vi "BioFeedback3(AudioInput+CircularBuffer).vi"() -> ()   [LabVIEW 2016]
uses:
  <vilib>/Analysis/5stat.llb/RMS (DBL).vi
  <vilib>/Analysis/baseanly.llb/Mean (DBL).vi
  <vilib>/Analysis/NI_AALBase.lvlib
  <vilib>/Analysis/NI_AALPro.lvlib
panel:
  out "Thermometer":dbl(slide) scale=0.0..0.07
  out "Circular Buffer Waveform\nData":waveform(dbl)(graph)
  out "Circular Buffer Waveform":waveform(dbl)[](graph)
  in  "bufferSize":dbl
  in  "Sample Duration":dbl
  out "filetered rms":waveform(dbl)(graph)
  out "filetered RMS Value 2":dbl
  out "RMS":waveform(dbl)(graph)
  out "RMS Value":dbl
  out "filtered":waveform(dbl)(graph)
  out "filtered + positivepeaks":waveform(dbl)(graph)
  out "Peaks Waveform (OLD)":waveform(dbl)(graph)
  out "Raw Audio\nWaveform":waveform(dbl)(graph)
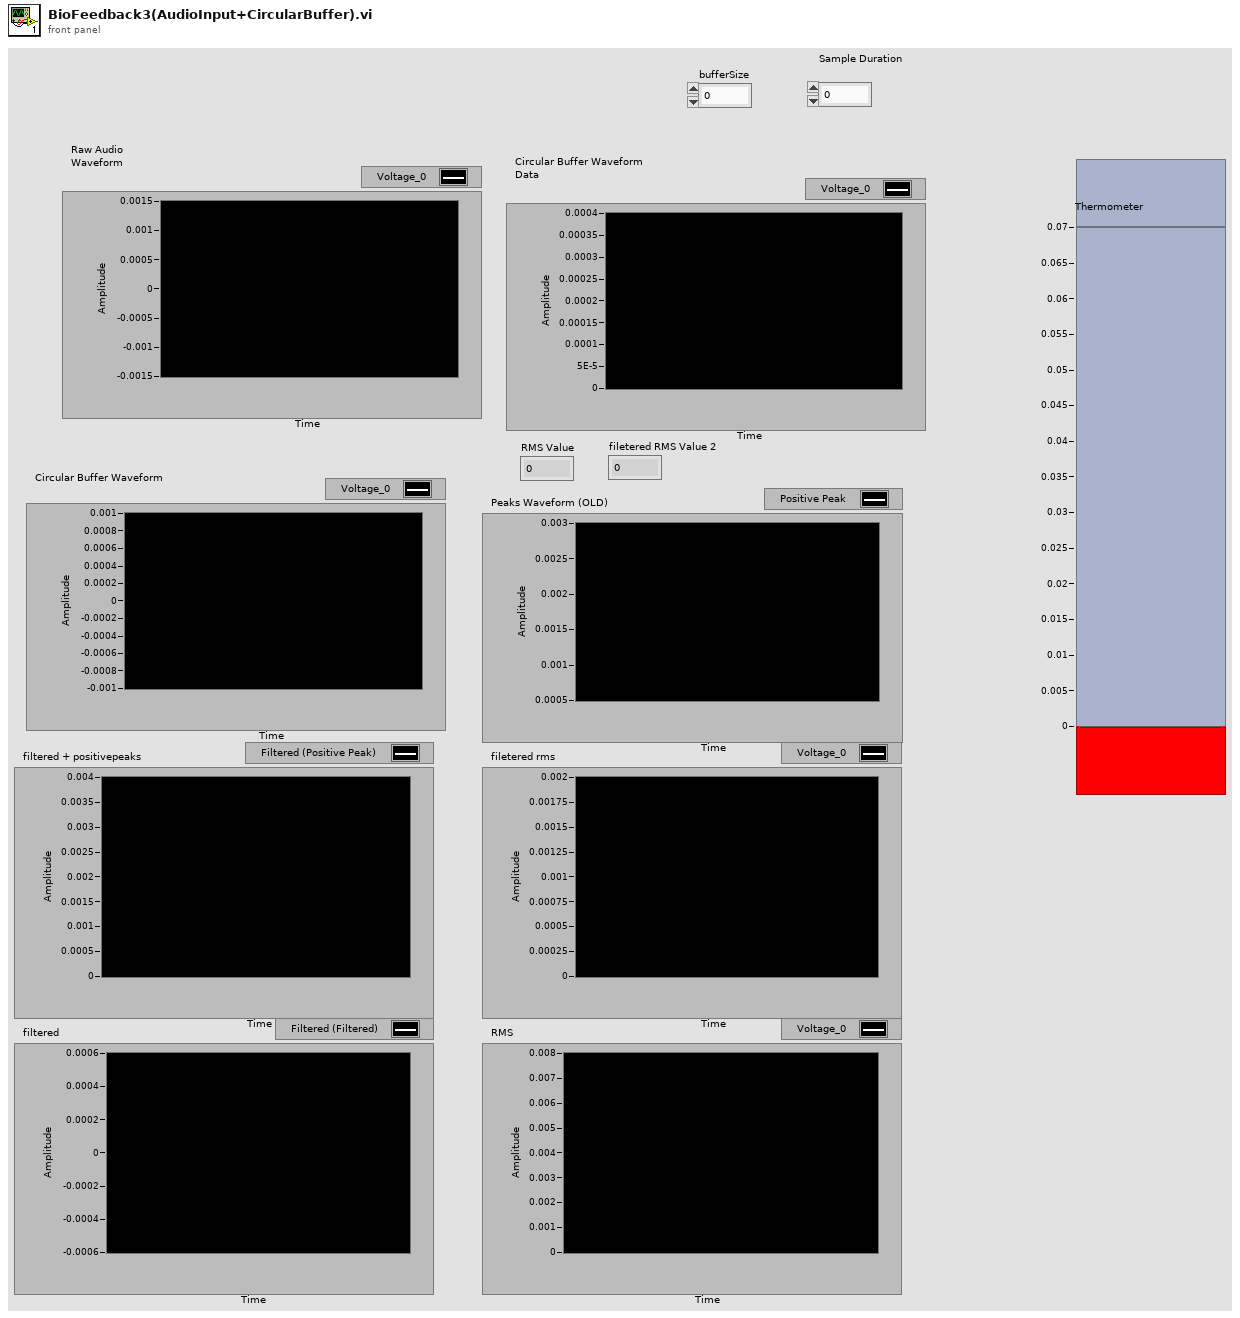
[diagram p1: front panel]
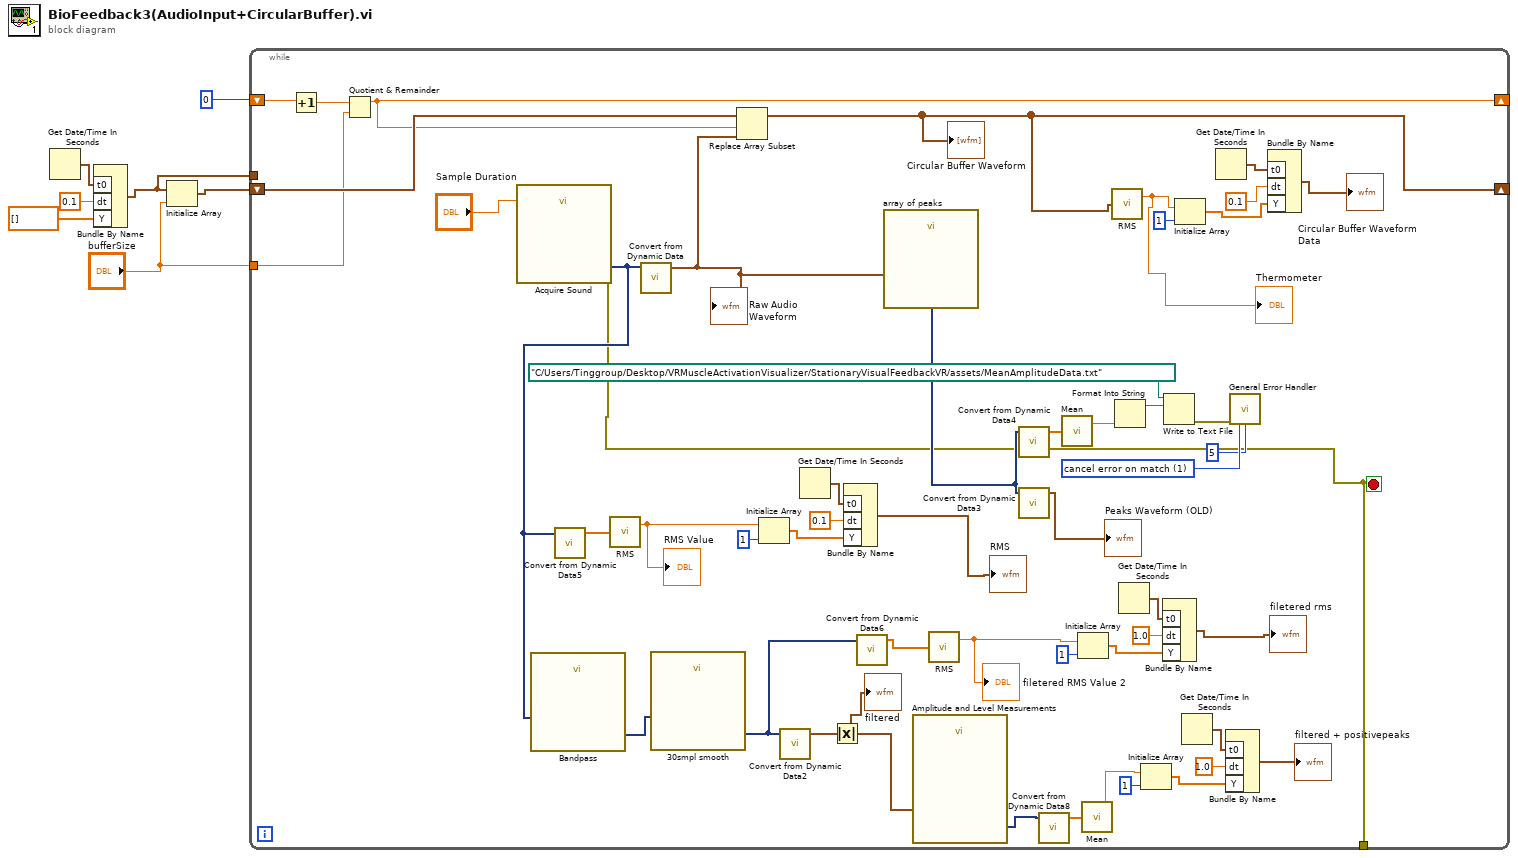
[diagram p0: block diagram]
diagram:
  n1 = Get Date/Time In Seconds() -> (seconds since 1Jan1904=w6:timestamp)
  n2 = Bundle By Name("t0"=w6, "dt"=0.1, "Y"=dbl[] []) -> (w1:waveform(dbl))  [unwired: 1 in]
  n3 = Initialize Array(w1, "bufferSize") -> (w4:waveform(dbl)[])
  n4 = while {
    tunnel: [w23] -> _
    shift-right: [w11] -> _
    shift-left: w4 -> [w18]
    shift-right: [w16] -> _
    shift-left: 0 -> [w20]
    tunnel: "bufferSize" -> [w15]
    tunnel: w1 -> [_]
    stop <- w23 stop-if-true
    w57 = 1 items=["no exception", "cancel error on match", "set error on match"] ("[exception action] (none:0)")
    n5 = Increment(x=w20) -> (x+1=w19:dbl)
    n6 = Quotient & Remainder(x=w19, y=w15) -> (x-y*floor(x/y)=w16:dbl)  [unwired: 1 out]
    n7 = call "Acquire Sound"("Duration (s)"="Sample Duration") -> ("Data"=w49:dynamicdata, "error out"=w23:errorcluster)  [unwired: 17 in]
    n8 = call "Bandpass"("Signal"=w49) -> ("Filtered Signal"=w50:dynamicdata)  [unwired: 9 in, 1 out]
    n9 = call "Convert from Dynamic Data5"("Dynamic Data Type"=w49) -> ("Array"=w48:dbl[])  [unwired: 3 in]
    n10 = call-poly <vilib>:"RMS.vi"("X"=w48) -> ("rms value"=w34:dbl)  [unwired: 1 out]
    "RMS Value" <- w34
    n11 = call "Convert from Dynamic Data"("Dynamic Data Type"=w49, "Channel"=w49) -> ("Waveform"=w17:waveform(dbl))  [unwired: 2 in]
    "Raw Audio\nWaveform" <- w17
    n12 = call "30smpl smooth"("Signal"=w50) -> ("Filtered Signal"=w38:dynamicdata)  [unwired: 9 in, 1 out]
    n13 = Replace Array Subset(array=w18, new element=w17, index=w16) -> (w11:waveform(dbl)[])
    "Circular Buffer Waveform" <- w11
    n14 = Initialize Array(w34, 1 ("dimension size")) -> (w46:dbl[])
    n15 = call "Convert from Dynamic Data2"("Dynamic Data Type"=w38) -> ("Waveform"=w39:waveform(dbl))  [unwired: 3 in]
    n16 = Get Date/Time In Seconds() -> (seconds since 1Jan1904=w52:timestamp)
    n17 = Absolute Value(x=w39) -> (abs(x)=w35:waveform(dbl))
    "filtered" <- w35
    n18 = Bundle By Name("t0"=w52, "dt"=0.1, "Y"=w46) -> (→"RMS":waveform(dbl))  [unwired: 1 in]
    n19 = call "Convert from Dynamic Data6"("Dynamic Data Type"=w38) -> ("Array"=w37:dbl[])  [unwired: 3 in]
    n20 = call "array of peaks"("Signals"=w17) -> ("Positive Peak"=w53:dynamicdata)  [unwired: 13 in, 1 out]
    n21 = call "Amplitude and Level Measurements"("Signals"=w35) -> ("Positive Peak"=w31:dynamicdata)  [unwired: 13 in, 1 out]
    n22 = call-poly <vilib>:"RMS.vi"("X"=w37) -> ("rms value"=w42:dbl)  [unwired: 1 out]
    "filetered RMS Value 2" <- w42
    n23 = call "Convert from Dynamic Data4"("Dynamic Data Type"=w53) -> ("Array"=w33:dbl[])  [unwired: 3 in]
    n24 = call "Convert from Dynamic Data3"("Dynamic Data Type"=w53) -> ("Waveform"=→"Peaks Waveform (OLD)":waveform(dbl))  [unwired: 3 in]
    n25 = call "Convert from Dynamic Data8"("Dynamic Data Type"=w31) -> ("Array"=w32:dbl[])  [unwired: 3 in]
    n26 = call-poly <vilib>:"Mean.vi"("X"=w33) -> ("mean"=w24:dbl)  [unwired: 1 out]
    n27 = Initialize Array(w42, 1 ("dimension size")) -> (w40:dbl[])
    n28 = call-poly <vilib>:"Mean.vi"("X"=w32) -> ("mean"=w26:dbl)  [unwired: 1 out]
    n29 = call-poly <vilib>:"RMS.vi"("X"=w11) -> ("rms value"=w8:dbl)  [unwired: 1 out]
    "Thermometer" <- w8
    n30 = Format Into String(w24) -> (resulting string=w55:string)  [unwired: 3 in, 1 out]
    n31 = Get Date/Time In Seconds() -> (seconds since 1Jan1904=w44:timestamp)
    n32 = Initialize Array(w26, 1 ("dimension size")) -> (w25:dbl[])
    n33 = Bundle By Name("t0"=w44, "dt"=1.0, "Y"=w40) -> (→"filetered rms":waveform(dbl))  [unwired: 1 in]
    n34 = Write to Text File(file (use dialog)=path "C:/Users/Tinggroup/Desktop/VRMuscleActivationVisualizer/StationaryVisualFeedbackVR/assets/MeanAmplitudeData.txt", text=w55) -> (error out=w58:errorcluster)  [unwired: 2 in, 2 out]
    n35 = Initialize Array(w8, 1 ("dimension size")) -> (w9:dbl[])
    n36 = Get Date/Time In Seconds() -> (seconds since 1Jan1904=w30:timestamp)
    n37 = Get Date/Time In Seconds() -> (seconds since 1Jan1904=w14:timestamp)
    n38 = Bundle By Name("t0"=w30, "dt"=1.0, "Y"=w25) -> (→"filtered + positivepeaks":waveform(dbl))  [unwired: 1 in]
    n39 = call <vilib>:"General Error Handler.vi"("error in (no error)"=w58, "[exception action] (none:0)"=w57, "[exception code]"=5) -> ()  [unwired: 8 in, 5 out]
    n40 = Bundle By Name("t0"=w14, "dt"=0.1, "Y"=w9) -> (→"Circular Buffer Waveform\nData":waveform(dbl))  [unwired: 1 in]
  }
